vi "FTW-CodeGen-Image.vi"(0 "State In":T1, 5 "XRef":refnum<vi>) -> (4 "Image":picture)   [LabVIEW 2012, in "FTW-JSON-Deserialize.xnode"]
uses:
  FTW-JSON-Deserialize.xnode
  FTW-CodeGen-State.ctl
panel:
  # "Inputs"
  # "Outputs"
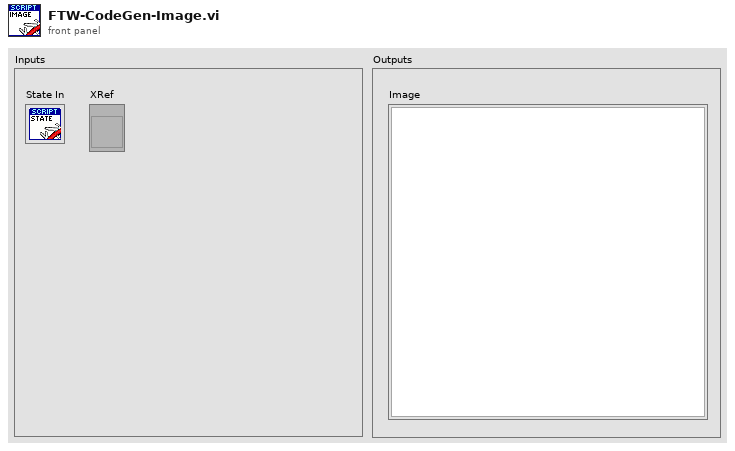
[diagram p1: front panel]
types:
  T1 = typedef "FTW-JSON-Deserialize.xnode/FTW-CodeGen-State.ctl" = cluster{"Dummy":string}
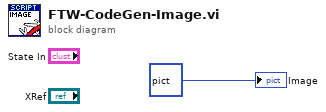
[diagram p0: block diagram]
diagram:
  "Image" <- picture bytes[3232] ("Image")
